vi "Test3v2.vi"() -> ()   [LabVIEW 2013]
panel:
  out "subarray":string[](array[string])
  out "index":i32
  out "Array":string[][](array[string])
  in  "stop":bool
  out "*(type *) &x":string
  out "size(s)":i32
  out "hex integer string":string[](array[string])
  in  "error in":errorcluster
  out "error out":errorcluster
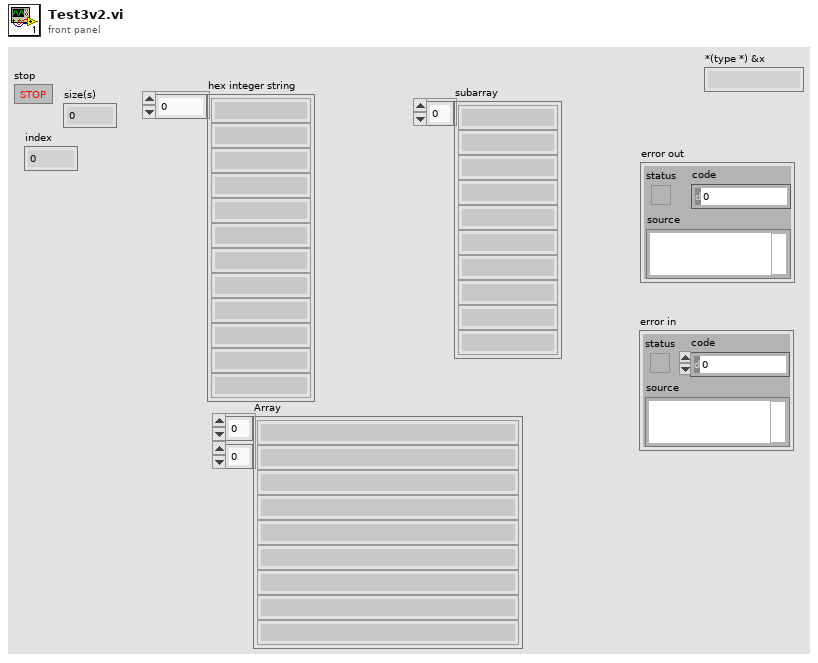
[diagram p1: front panel]
types:
  T1 = enum16{"big-endian, network order", "native, host order", "little-endian"}
  T2 = enum16{"open", "replace", "create", "open or create", "replace or create", "replace or create with confirmation"}
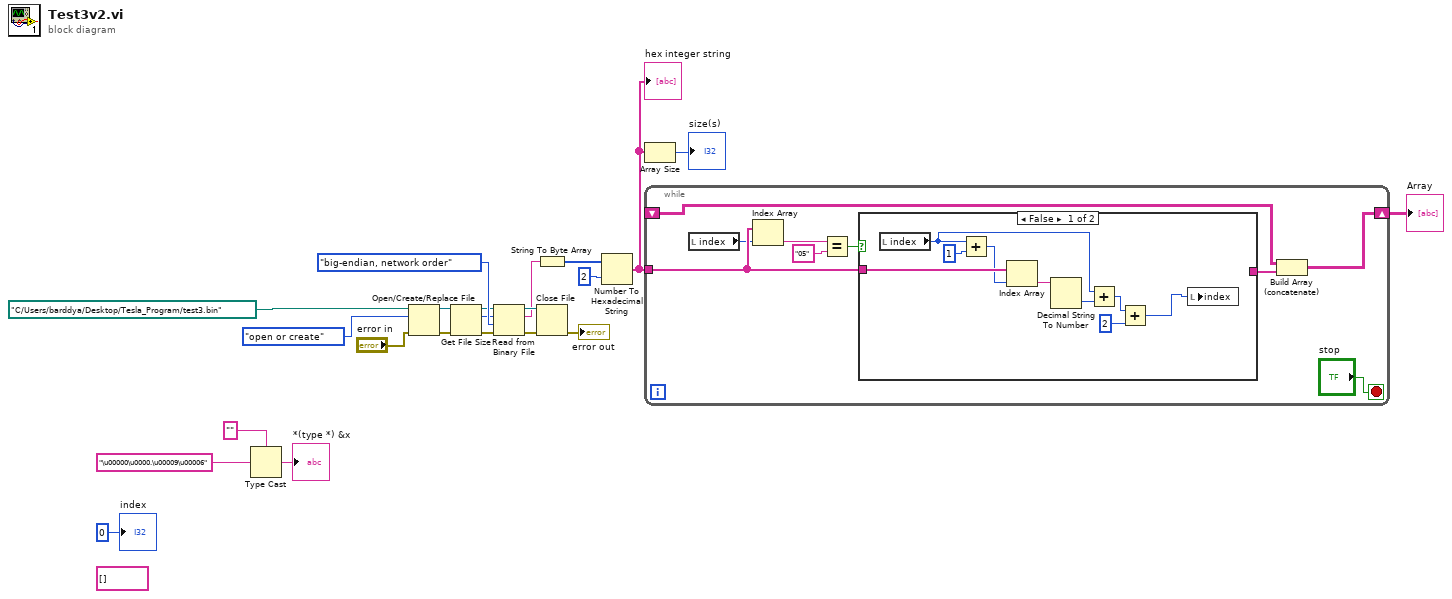
[diagram p0: block diagram]
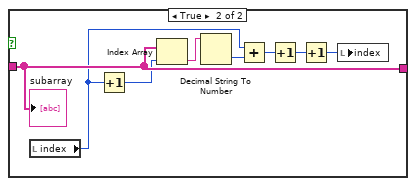
[diagram p2: hidden frame]
diagram:
  (unwired) string[] [] ("subarray")
  n1 = Type Cast(type="", x="\u00000\u0000.\u00009\u00006") -> (*(type *) &x=→"*(type *) &x":string)
  n2 = Open/Create/Replace File(file path (use dialog)=path "C:/Users/barddya/Desktop/Tesla_Program/test3.bin", error in="error in", operation (0:open)=T2."open or create") -> (refnum out=w15:refnum<file>, error out=w13:errorcluster)  [unwired: 3 in, 1 out]
  n3 = Get File Size(file=w15, error in=w13) -> (refnum out=w14:refnum<file>, size (in bytes)=w11:i64, 0:w12:errorcluster)
  n4 = Read from Binary File(8:w12, 9:T1."big-endian, network order" ("byte order (0:big-endian, network order)"), 10:w11, 11:w14) -> (0:w18:errorcluster, 2:w10:string, 3:w16:refnum<file>)  [unwired: 2 in, 1 out]
  n5 = String To Byte Array(string=w10) -> (unsigned byte array=w9:u8[])
  n6 = Close File(refnum=w16, error in=w18) -> (error out=→"error out":errorcluster)  [unwired: 1 out]
  n7 = Number To Hexadecimal String(1:2, 2:w9) -> (0:w3:string[])
  "hex integer string" <- w3
  n8 = Array Size(array=w3) -> (size(s)=→"size(s)":i32)
  n9 = while {
    shift-right: [w31] -> w2
    shift-left: _ -> [w30]
    tunnel: w3 -> [w26]
    stop <- "stop" stop-if-true
    n10 = local read "index"() -> (w23:i32)
    n11 = Index Array(array=w26, index=w23) -> (element=w29:string)
    n12 = Equal?(x=w29, y="05") -> (x = y?=w27:bool)
    n13 = case shown="False" w27 {
      tunnel: w26 -> [w38 w46]
      tunnel: [_ w46] -> w25
      frame False {
        n14 = local read "index"() -> (w35:i32)
        n15 = Add(x=w35, y=1) -> (x+y=w36:i32)
        n16 = Index Array(array=w38, index=w36) -> (element=w40:string)
        n17 = Decimal String To Number(string=w40) -> (number=w39:i32)  [unwired: 2 in, 1 out]
        n18 = Add(x=w35, y=w39) -> (x+y=w34:i32)
        n19 = Add(x=w34, y=2) -> (x+y=w32:i32)
        n20 = local write "index"(w32) -> ()
      }
      frame True {
        n21 = local read "index"() -> (w43:i32)
        n22 = Increment(x=w43) -> (x+1=w45:i32)
        n23 = Index Array(array=w46, index=w45) -> (element=w48:string)
        n24 = Decimal String To Number(string=w48) -> (number=w47:i32)  [unwired: 2 in, 1 out]
        n25 = Add(x=w43, y=w47) -> (x+y=w44:i32)
        n26 = Increment(x=w44) -> (x+1=w42:i32)
        n27 = Increment(x=w42) -> (x+1=w41:i32)
        n28 = local write "index"(w41) -> ()
        "subarray" <- w46
      }
    }
    n29 = Build Array (concatenate)(w30, w25) -> (w31:string[][])
  }
  "Array" <- w2
  "index" <- 0
